vi "Obtain Session.vi"(2 "TS License Type (Operator)":T1, 7 "Debug Daemon (Dev Only)":bool, 11 "error in (no error)":errorcluster, 13 "Error to Create? (F)":bool) -> (3 "Acquired License":T1, 4 "Session Handle":T2, 15 "error out":errorcluster)   [LabVIEW 2020, in "TSS.lvlib" / "Engine.lvclass"]
doc: "This function initializes the measurement\n\nPass the function a name to obtain an active measurement handle"
uses:
  Engine.lvclass
  Typedefs/Session Handle.ctl
  C:/Program Files (x86)/National Instruments/LabVIEW 2020/user.lib/_Session Fwk/Session - Root.lvclass
  TS License Type.ctl
  Engine.lvclass/Engine.ctl
  Get TS License Type.vi
  <userlib>/_Session Fwk/Session - Root.lvclass
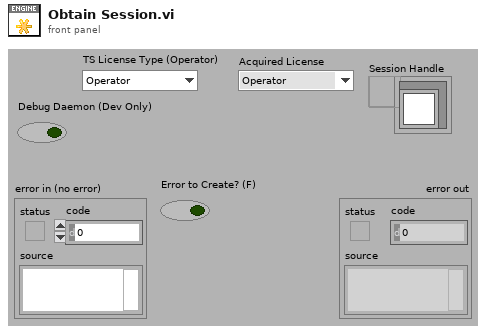
[diagram p1: front panel]
types:
  T1 = typedef "TSS.lvlib/Engine.lvclass/TS License Type.ctl" = enum16{"Operator", "CustomEditor", "SequenceEditor"}
  T2 = typedef "TSS.lvlib/Engine.lvclass/Session Handle.ctl" = refnum<data-value>
  T3 = enum32{"invalid app kind", "Development System", "Run Time System", "Student Edition", "Embedded LabVIEW", "Evaluation", "Custom"}
  T4 = typedef "Session - Root.lvclass/Session Handle.ctl" = refnum<data-value>
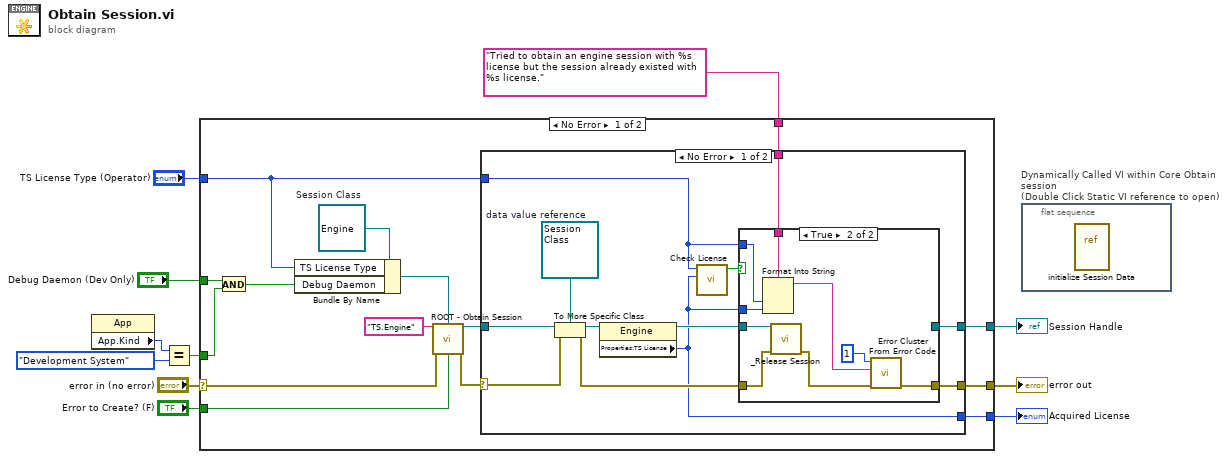
[diagram p0: block diagram]
diagram:
  n1 = property class="App"() -> ("App.Kind"=w5:T3)  [unwired: 2 in, 2 out]
  n2 = Equal?(x=w5, y=T3."Development System") -> (x = y?=w3:bool)
  n3 = case shown="No Error" "error in (no error)" {
    selector: "error in (no error)" -> [w26 w51]
    tunnel: [w19 w51] -> w10
    tunnel: [w20 _] -> w9
    tunnel: "TS License Type (Operator)" -> [w18 _]
    tunnel: "Tried to obtain an engine session with %s license but the session already existed with %s license." -> [w17 _]
    tunnel: "Error to Create? (F)" -> [w16 _]
    tunnel: w3 -> [w14 _]
    tunnel: "Debug Daemon (Dev Only)" -> [w13 _]
    tunnel: [w12 _] -> w1
    frame No Error {
      w22 = refnum<class "Engine.lvclass"> refnum  # Session Class
      n4 = And(x=w13, y=w14) -> (x .and. y?=w15:bool)
      n5 = Bundle By Name(cluster=w22, "TS License Type"=w18, "Debug Daemon"=w15) -> (w21:refnum<class "Engine.lvclass">)
      n6 = call <userlib>:"ROOT - Obtain Session.vi"("Session Name ()"="TS.Engine", "OBJ - Session"=w21, "error in (no error)"=w26, "Error to Create? (F)"=w16) -> ("Session Handle"=w24:T4, "error out"=w25:errorcluster)  [unwired: 9 in, 1 out]
      n7 = case shown="No Error" w25 {
        selector: w25 -> [w38 w50]
        tunnel: w24 -> [w37 _]
        tunnel: [w32 _] -> w20
        tunnel: [w31 w50] -> w19
        tunnel: w18 -> [w29 _]
        tunnel: w17 -> [w30 _]
        tunnel: [w27 _] -> w12
        frame No Error {
          w36 = refnum<data-value> refnum  # data value reference
          n8 = To More Specific Class(target class=w36, reference=w37, error in=w38) -> (specific class reference=w35:refnum<data-value>, error out=w34:errorcluster)
          n9 = property class="Engine"(reference=w35) -> (reference out=w33:refnum<data-value>, "Properties:TS License"=w27:T1)  [unwired: 1 in, 1 out]
          n10 = call "Check License.vi"("Existing License"=w27, "Requested License"=w29) -> ("Invalid?"=w28:bool)  [unwired: 9 in]
          n11 = case shown="True" w28 {
            tunnel: w34 -> [w39 w42]
            tunnel: w33 -> [w40 w43]
            tunnel: [w40 _] -> w32
            tunnel: [w39 w49] -> w31
            tunnel: w27 -> [_ w46]
            tunnel: w29 -> [_ w45]
            tunnel: w30 -> [_ w47]
            frame False {
            }
            frame True {
              n12 = Format Into String(format string=w47, w45, w46) -> (resulting string=w44:string)  [unwired: 2 in, 1 out]
              n13 = call "_Release Session.vi"("Session Handle"=w43, "error in (no error)"=w42) -> ("error out"=w41:errorcluster)  [unwired: 13 in]
              n14 = call <vilib>:"Error Cluster From Error Code.vi"("error in (no error)"=w41, "error message (\"\")"=w44, "error code (0)"=1) -> ("error out"=w49:errorcluster)  [unwired: 6 in]
            }
          }
        }
        frame Error {
        }
      }
    }
    frame Error {
    }
  }
  "error out" <- w10
  "Session Handle" <- w9
  "Acquired License" <- w1
  n15 = flat-sequence "Dynamically Called VI within Core Obtain session\n(Double Click Static VI reference to open)" {
    frame #0 {
      n16 = vi-ref "initialize Session Data.vi"() -> ()  [unwired: 1 out]
    }
  }
